vi "main.vi"() -> ()   [LabVIEW 2016]
uses:
  <vilib>/FPGAPlugInAG/myRIO-1900/niLvFpga_Open_myRIO-1900.vi
  <vilib>/rvi/interface/common/dynamic/niFpgaDynamicAddResources.vi
  <vilib>/Utility/error.llb/Error Cluster From Error Code.vi
  <vilib>/rvi/errors/niLvFpgaAdjustHostInterfaceError.vi
  <vilib>/FPGAPlugInAG/Dynamic/niLvFpga_Close_Dynamic.vi
  <vilib>/rvi/interface/nirviOpenFPGA/nirviOpenFPGA.xnode
  FPGA Bitfiles/Musicbox_FPGATarget_soundctrl_6-HSKECpU5c.lvbitx
  sound_ctrl.vi
  <vilib>/rvi/interface/nirviReadWriteControl/nirviReadWriteControl.xnode
  <vilib>/rvi/interface/nirviCloseFPGA/nirviCloseFPGA.xnode
  NiFpgaLv.dll
  <vilib>/rvi/interface/Simulation/niFpgaSimulationCallBeginRW.vi
panel:
  out "Chosen frequency":dbl
  in  "Combine frequencies":bool
  out "Saved Frequency":dbl
  in  "Add Button":bool
  out "Current Frequency":dbl
  out "Volume":dbl
  out "flag":bool
  out "index":dbl
  out "z":dbl
  out "y":dbl
  out "x":dbl
  in  "stop":bool
  out "1":string
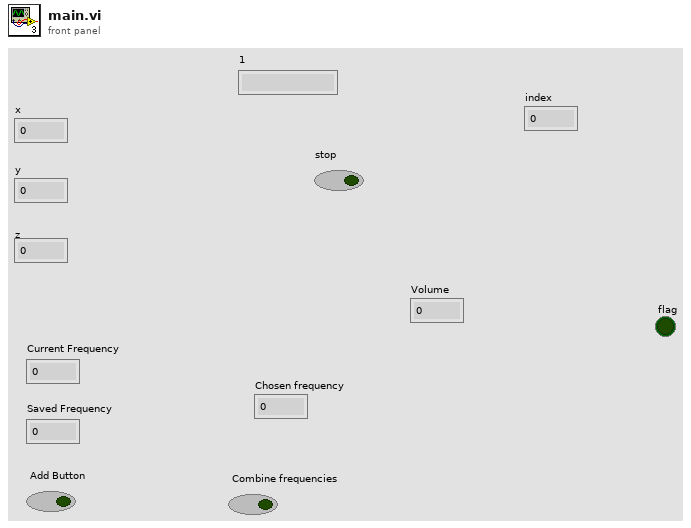
[diagram p1: front panel]
types:
  T1 = enum16{"1", "volume_+", "volume_-", "frequency+", "frequency-", "note1_selec", "note2_selec", "idle 2", "idle 3"}
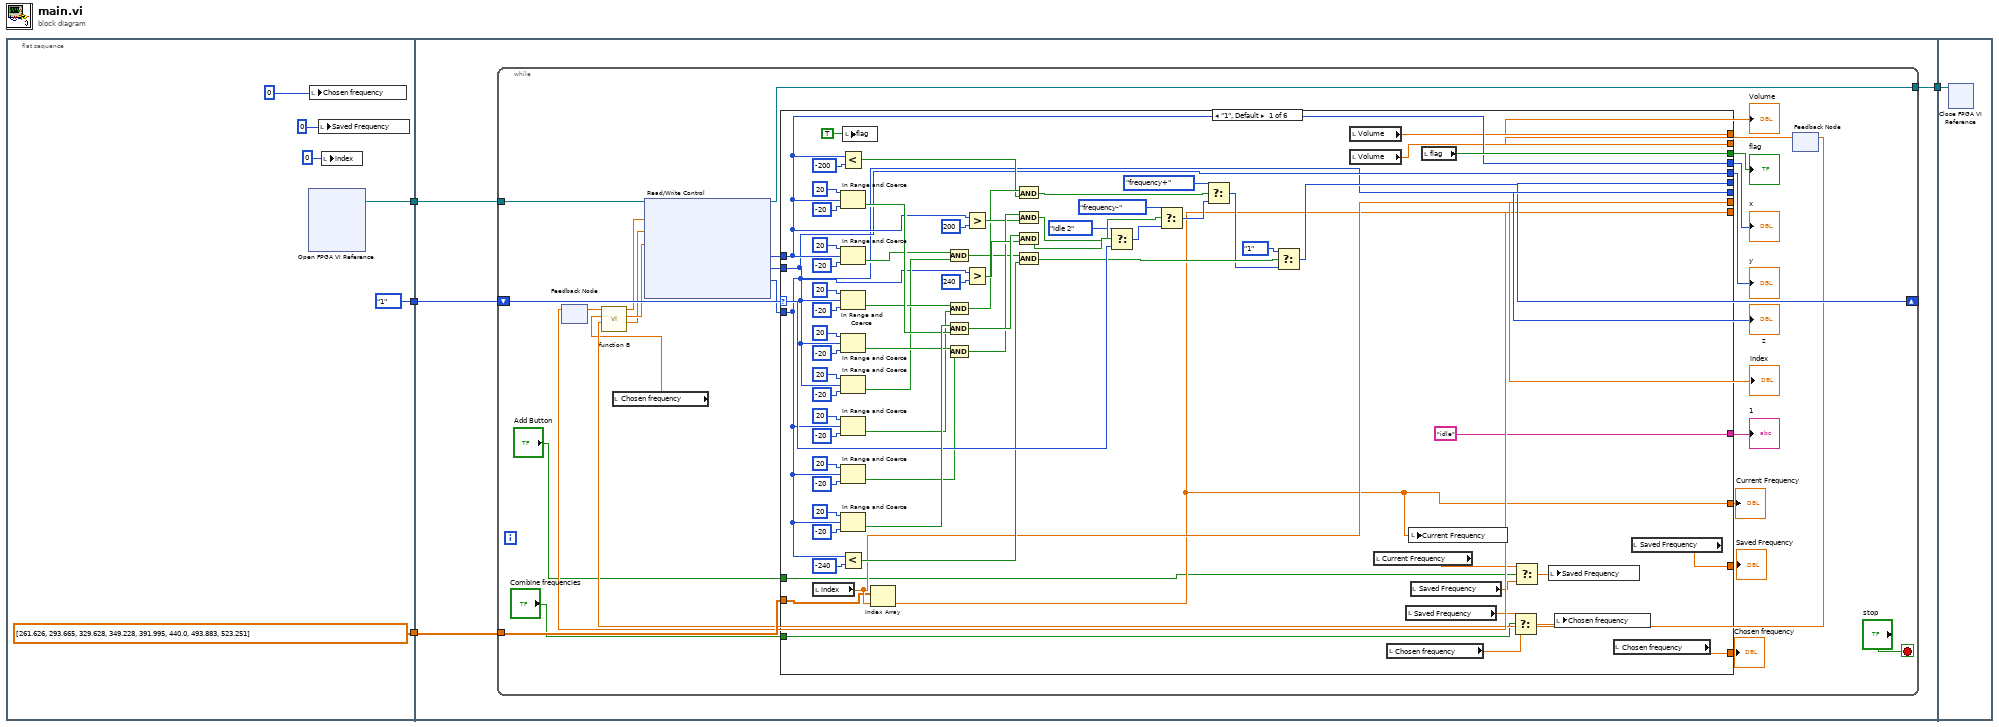
[diagram p0: block diagram]
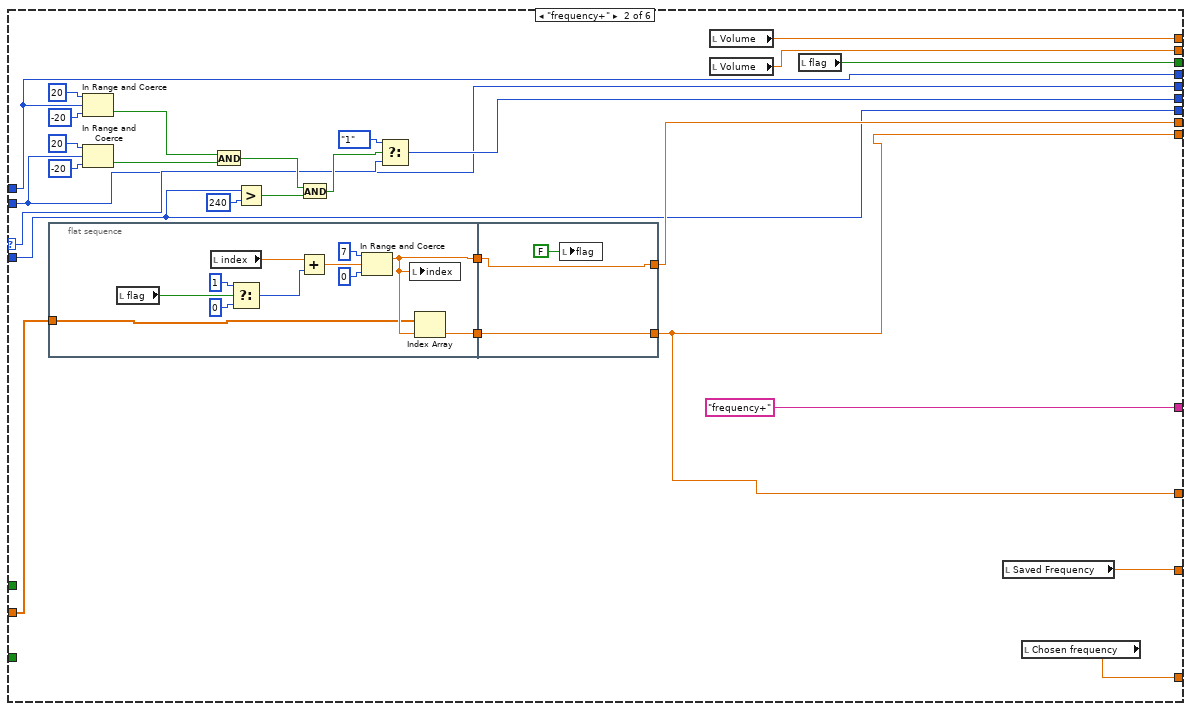
[diagram p2: hidden frame]
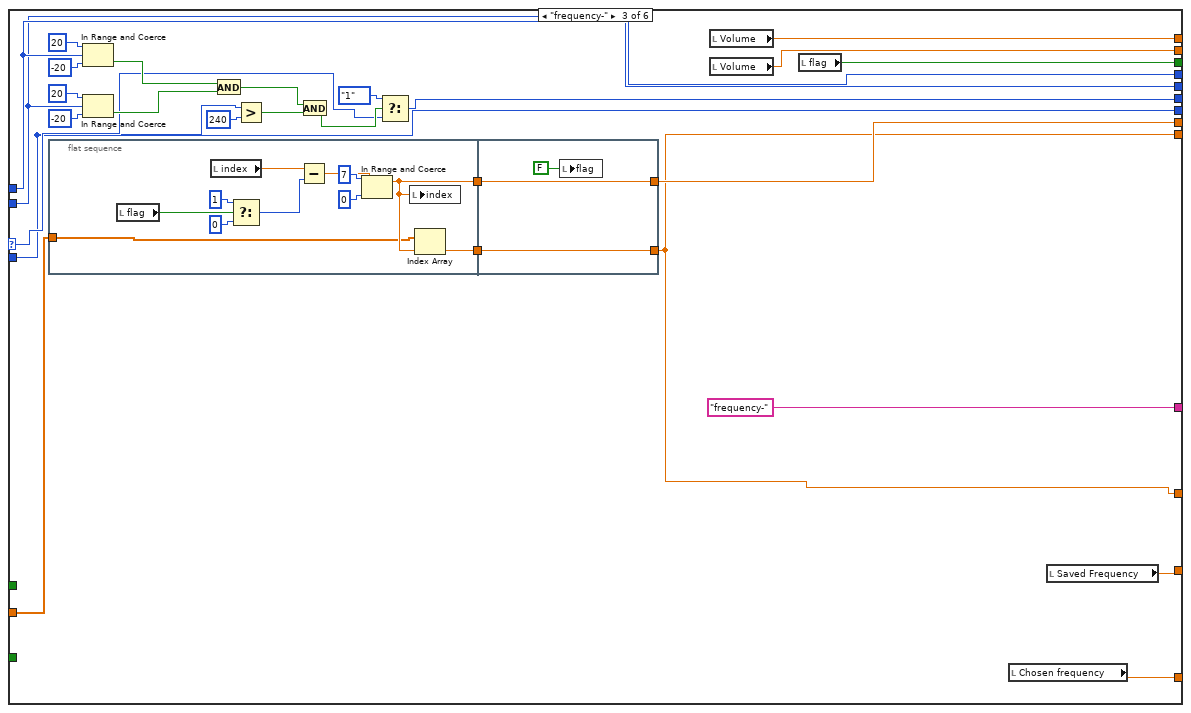
[diagram p3: hidden frame]
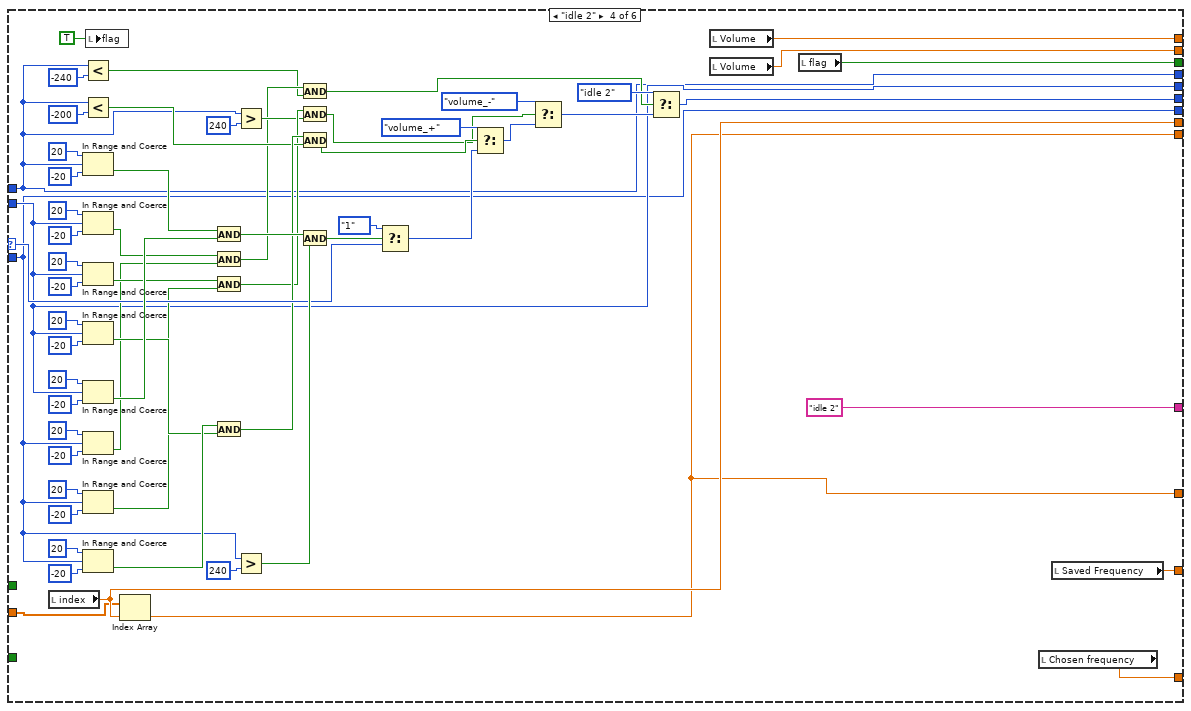
[diagram p4: hidden frame]
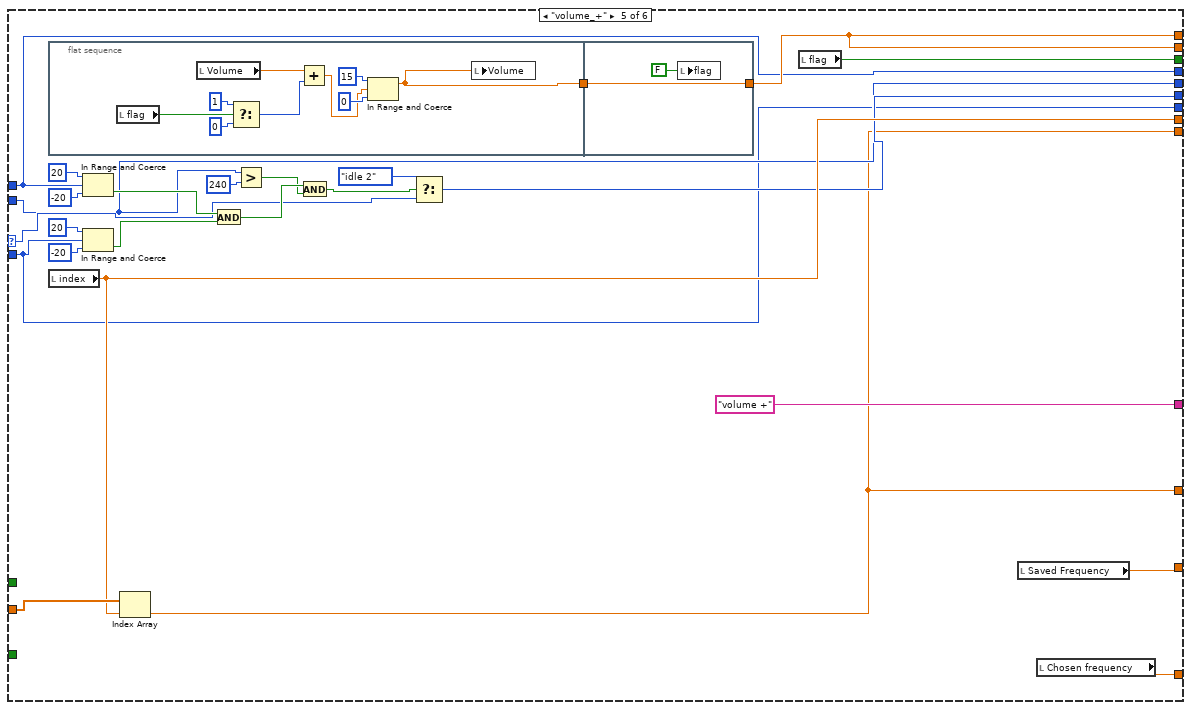
[diagram p5: hidden frame]
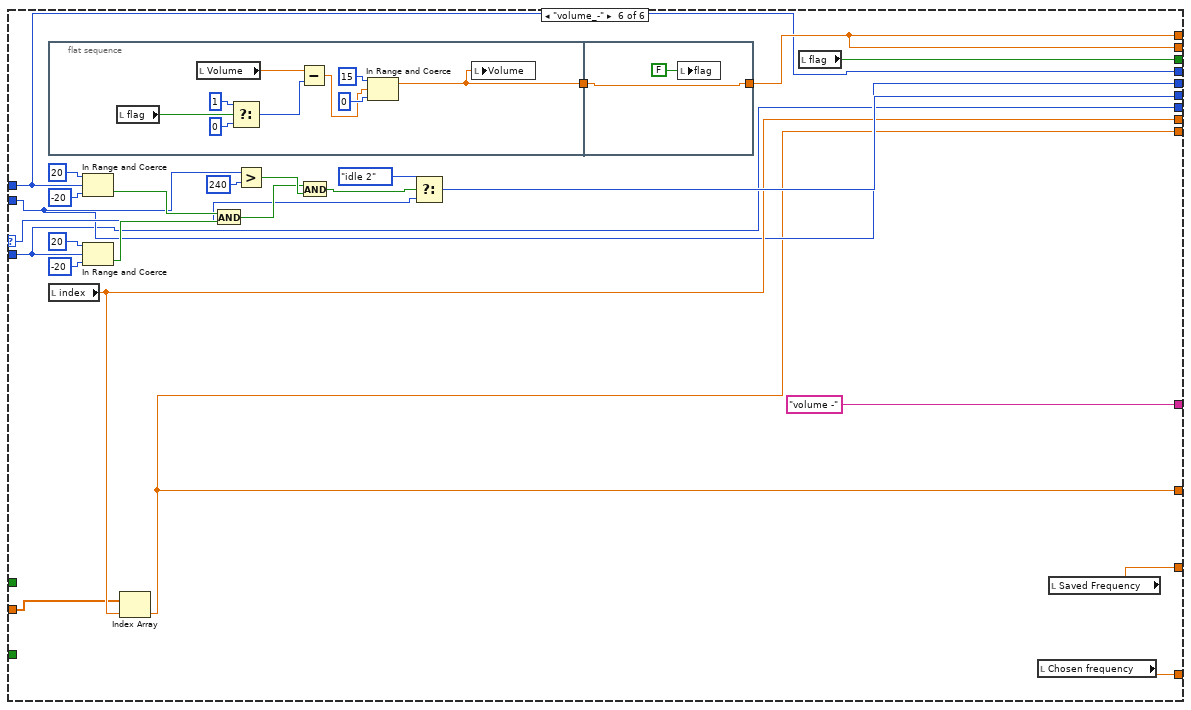
[diagram p6: hidden frame]
diagram:
  n1 = flat-sequence {
    tunnel: [w9] -> w3
    tunnel: [T1."1"] -> w2
    tunnel: [dbl[] [261.626, 293.665, 329.628, 349.228, 391.995, 440.0, 493.883, 523.251]] -> w1
    tunnel: [w14] -> w4
    tunnel: w3 -> [w13]
    tunnel: w2 -> [w12]
    tunnel: w1 -> [w11]
    tunnel: w4 -> [w329]
    frame #0 {
      n2 = xnode "Open FPGA VI Reference"() -> ("FPGA VI Reference Out"=w9:refnum<k20>)  [unwired: 2 in, 1 out]
      n3 = local write "Chosen frequency"(0) -> ()
      n4 = local write "Saved Frequency"(0) -> ()
      n5 = local write "index"(0) -> ()
    }
    frame #1 {
      n6 = while {
        shift-right: [w36] -> _
        shift-left: w12 -> [w37]
        tunnel: [w27] -> w14
        tunnel: w13 -> [w26]
        tunnel: w11 -> [w25]
        stop <- "stop" stop-if-true
        n7 = feedback #1() -> (w23:dbl)  [unwired: 1 in]
        n8 = local read "Chosen frequency"() -> (w16:dbl)
        n9 = feedback #2() -> (w20:dbl)  [unwired: 1 in]
        n10 = call "function B.vi"("frequency 1"=w23, "frequency 2"=w16, "volume"=w20) -> ("Frequency Indicator"=w30:dbl, "Frequency Indicator 2"=w29:dbl, "Volume Indicator"=w28:dbl)  [unwired: 5 in]
        n11 = xnode ("Read/Write Control")("FPGA VI Reference In"=w26, "frequency (periods/tick)"=w30, "Volume"=w28, "frequency (periods/tick) 2"=w29) -> ("FPGA VI Reference Out"=w27:refnum<k20>, "AccelerationX"=w33:i16, "AccelerationY"=w32:i16, "AccelerationZ"=w31:i16)  [unwired: 2 in, 1 out]
        n12 = case shown="\"1\", Default" w37 {
          selector: w37 -> [w101 w125 w166 w246 w262 w301]
          tunnel: ["idle" "frequency+" "frequency-" "idle 2" "volume +" "volume -"] -> w42
          tunnel: [w60 w120 w161 w199 w264 w299] -> w40
          tunnel: [w59 w119 w160 w205 w261 w297] -> w39
          tunnel: [w58 w118 w159 w198 w260 w296] -> w38
          tunnel: [w64 w123 w164 w208 w263 w304] -> w36
          tunnel: [w57 w138 w177 w204 w278 w303] -> w35
          tunnel: [w62 w122 w163 w207 w277 w298] -> w34
          tunnel: w33 -> [w60 w120 w161 w199 w264 w299]
          tunnel: w32 -> [w59 w119 w160 w205 w261 w297]
          tunnel: w31 -> [w58 w118 w159 w198 w260 w296]
          tunnel: w25 -> [w56 w121 w162 w203 w279 w302]
          tunnel: [w53 w115 w156 w197 w259 w295] -> w24
          tunnel: [w55 w116 w158 w201 w280 w300] -> w22
          tunnel: [w54 w117 w157 w202 w280 w300] -> w21
          tunnel: [w53 w115 w156 w197 w259 w295] -> w19
          tunnel: [w49 w114 w155 w196 w258 w294] -> _
          tunnel: "Add Button" -> [w48 _ _ _ _ _]
          tunnel: "Combine frequencies" -> [w47 _ _ _ _ _]
          tunnel: [w44 w113 w154 w195 w257 w293] -> w15
          frame "1", Default {
            n13 = local read "index"() -> (w57:dbl)
            n14 = Less?(x=w60, y=-200) -> (x < y?=w83:bool)
            n15 = In Range and Coerce(upper limit=20, x=w60, lower limit=-20) -> (In Range?=w105:bool)  [unwired: 1 out]
            n16 = In Range and Coerce(upper limit=20, x=w60, lower limit=-20) -> (In Range?=w72:bool)  [unwired: 1 out]
            n17 = In Range and Coerce(upper limit=20, x=w59, lower limit=-20) -> (In Range?=w86:bool)  [unwired: 1 out]
            n18 = In Range and Coerce(upper limit=20, x=w59, lower limit=-20) -> (In Range?=w96:bool)  [unwired: 1 out]
            n19 = In Range and Coerce(upper limit=20, x=w59, lower limit=-20) -> (In Range?=w71:bool)  [unwired: 1 out]
            n20 = In Range and Coerce(upper limit=20, x=w58, lower limit=-20) -> (In Range?=w85:bool)  [unwired: 1 out]
            n21 = In Range and Coerce(upper limit=20, x=w58, lower limit=-20) -> (In Range?=w95:bool)  [unwired: 1 out]
            n22 = In Range and Coerce(upper limit=20, x=w58, lower limit=-20) -> (In Range?=w106:bool)  [unwired: 1 out]
            n23 = Less?(x=w58, y=-240) -> (x < y?=w69:bool)
            n24 = local write "flag"(TRUE) -> ()
            n25 = Index Array(array=w56, index=w57) -> (element=w53:dbl)
            n26 = And(x=w72, y=w71) -> (x .and. y?=w70:bool)
            n27 = And(x=w86, y=w85) -> (x .and. y?=w84:bool)
            n28 = And(x=w106, y=w105) -> (x .and. y?=w104:bool)
            n29 = And(x=w96, y=w95) -> (x .and. y?=w94:bool)
            n30 = Greater?(x=w60, y=200) -> (0:w93:bool)
            n31 = Greater?(x=w59, y=240) -> (0:w103:bool)
            n32 = And(x=w84, y=w83) -> (x .and. y?=w81:bool)
            n33 = And(x=w94, y=w93) -> (x .and. y?=w92:bool)
            n34 = And(x=w104, y=w103) -> (x .and. y?=w102:bool)
            n35 = And(x=w70, y=w69) -> (x .and. y?=w66:bool)
            n36 = Select(t=T1."idle 2", s=w102, f=w101) -> (s? t:f=w91:T1)
            n37 = Select(t=T1."frequency-", s=w92, f=w91) -> (s? t:f=w80:T1)
            n38 = Select(t=T1."frequency+", s=w81, f=w80) -> (s? t:f=w65:T1)
            n39 = Select(t=T1."1", s=w66, f=w65) -> (s? t:f=w64:T1)
            n40 = local read "Volume"() -> (w55:dbl)
            n41 = local read "Volume"() -> (w54:dbl)
            n42 = local read "Current Frequency"() -> (w51:dbl)
            n43 = local read "Chosen frequency"() -> (w43:dbl)
            n44 = local read "Saved Frequency"() -> (w46:dbl)
            n45 = local write "Current Frequency"(w53) -> ()
            n46 = local read "Saved Frequency"() -> (w52:dbl)
            n47 = local read "flag"() -> (w62:bool)
            n48 = Select(t=w46, s=w47, f=w43) -> (s? t:f=w45:dbl)
            n49 = Select(t=w51, s=w48, f=w52) -> (s? t:f=w50:dbl)
            n50 = local write "Saved Frequency"(w50) -> ()
            n51 = local write "Chosen frequency"(w45) -> ()
            n52 = local read "Chosen frequency"() -> (w44:dbl)
            n53 = local read "Saved Frequency"() -> (w49:dbl)
          }
          frame "frequency+" {
            n54 = flat-sequence {
              tunnel: [w150] -> w137
              tunnel: [w141] -> w136
              tunnel: w121 -> [w140]
              tunnel: [w152] -> w138
              tunnel: [w153] -> w115
              tunnel: w137 -> [w153]
              tunnel: w136 -> [w152]
              frame #0 {
                n55 = local read "flag"() -> (w145:bool)
                n56 = local read "index"() -> (w149:dbl)
                n57 = Select(t=1, s=w145, f=0) -> (s? t:f=w146:i32)
                n58 = Add(x=w149, y=w146) -> (x+y=w142:dbl)
                n59 = In Range and Coerce(upper limit=7, x=w142, lower limit=0) -> (coerced(x)=w141:dbl)  [unwired: 1 out]
                n60 = local write "index"(w141) -> ()
                n61 = Index Array(array=w140, index=w141) -> (element=w150:dbl)
              }
              frame #1 {
                n62 = local write "flag"(FALSE) -> ()
              }
            }
            n63 = In Range and Coerce(upper limit=20, x=w120, lower limit=-20) -> (In Range?=w130:bool)  [unwired: 1 out]
            n64 = In Range and Coerce(upper limit=20, x=w119, lower limit=-20) -> (In Range?=w129:bool)  [unwired: 1 out]
            n65 = And(x=w130, y=w129) -> (x .and. y?=w128:bool)
            n66 = Greater?(x=w118, y=240) -> (0:w127:bool)
            n67 = And(x=w128, y=w127) -> (x .and. y?=w126:bool)
            n68 = Select(t=T1."1", s=w126, f=w125) -> (s? t:f=w123:T1)
            n69 = local read "Volume"() -> (w116:dbl)
            n70 = local read "Volume"() -> (w117:dbl)
            n71 = local read "flag"() -> (w122:bool)
            n72 = local read "Saved Frequency"() -> (w114:dbl)
            n73 = local read "Chosen frequency"() -> (w113:dbl)
          }
          frame "frequency-" {
            n74 = flat-sequence {
              tunnel: [w191] -> w179
              tunnel: [w182] -> w178
              tunnel: w162 -> [w181]
              tunnel: [w193] -> w177
              tunnel: [w194] -> w156
              tunnel: w179 -> [w194]
              tunnel: w178 -> [w193]
              frame #0 {
                n75 = local read "flag"() -> (w188:bool)
                n76 = local read "index"() -> (w187:dbl)
                n77 = Select(t=1, s=w188, f=0) -> (s? t:f=w186:i32)
                n78 = Subtract(x=w187, y=w186) -> (x-y=w183:dbl)
                n79 = In Range and Coerce(upper limit=7, x=w183, lower limit=0) -> (coerced(x)=w182:dbl)  [unwired: 1 out]
                n80 = local write "index"(w182) -> ()
                n81 = Index Array(array=w181, index=w182) -> (element=w191:dbl)
              }
              frame #1 {
                n82 = local write "flag"(FALSE) -> ()
              }
            }
            n83 = In Range and Coerce(upper limit=20, x=w161, lower limit=-20) -> (In Range?=w171:bool)  [unwired: 1 out]
            n84 = In Range and Coerce(upper limit=20, x=w160, lower limit=-20) -> (In Range?=w170:bool)  [unwired: 1 out]
            n85 = And(x=w171, y=w170) -> (x .and. y?=w169:bool)
            n86 = Greater?(x=w159, y=240) -> (0:w168:bool)
            n87 = And(x=w169, y=w168) -> (x .and. y?=w167:bool)
            n88 = Select(t=T1."1", s=w167, f=w166) -> (s? t:f=w164:T1)
            n89 = local read "Volume"() -> (w158:dbl)
            n90 = local read "Volume"() -> (w157:dbl)
            n91 = local read "flag"() -> (w163:bool)
            n92 = local read "Chosen frequency"() -> (w154:dbl)
            n93 = local read "Saved Frequency"() -> (w155:dbl)
          }
          frame "idle 2" {
            n94 = local read "index"() -> (w204:dbl)
            n95 = Less?(x=w199, y=-240) -> (x < y?=w213:bool)
            n96 = Less?(x=w199, y=-200) -> (x < y?=w237:bool)
            n97 = In Range and Coerce(upper limit=20, x=w199, lower limit=-20) -> (In Range?=w251:bool)  [unwired: 1 out]
            n98 = In Range and Coerce(upper limit=20, x=w205, lower limit=-20) -> (In Range?=w216:bool)  [unwired: 1 out]
            n99 = In Range and Coerce(upper limit=20, x=w205, lower limit=-20) -> (In Range?=w227:bool)  [unwired: 1 out]
            n100 = In Range and Coerce(upper limit=20, x=w205, lower limit=-20) -> (In Range?=w239:bool)  [unwired: 1 out]
            n101 = In Range and Coerce(upper limit=20, x=w205, lower limit=-20) -> (In Range?=w250:bool)  [unwired: 1 out]
            n102 = In Range and Coerce(upper limit=20, x=w198, lower limit=-20) -> (In Range?=w215:bool)  [unwired: 1 out]
            n103 = In Range and Coerce(upper limit=20, x=w198, lower limit=-20) -> (In Range?=w226:bool)  [unwired: 1 out]
            n104 = In Range and Coerce(upper limit=20, x=w198, lower limit=-20) -> (In Range?=w240:bool)  [unwired: 1 out]
            n105 = local write "flag"(TRUE) -> ()
            n106 = Index Array(array=w203, index=w204) -> (element=w197:dbl)
            n107 = And(x=w251, y=w250) -> (x .and. y?=w249:bool)
            n108 = And(x=w216, y=w215) -> (x .and. y?=w214:bool)
            n109 = And(x=w227, y=w226) -> (x .and. y?=w225:bool)
            n110 = And(x=w240, y=w239) -> (x .and. y?=w238:bool)
            n111 = Greater?(x=w199, y=240) -> (0:w224:bool)
            n112 = Greater?(x=w198, y=240) -> (0:w248:bool)
            n113 = And(x=w214, y=w213) -> (x .and. y?=w210:bool)
            n114 = And(x=w225, y=w224) -> (x .and. y?=w222:bool)
            n115 = And(x=w238, y=w237) -> (x .and. y?=w234:bool)
            n116 = And(x=w249, y=w248) -> (x .and. y?=w247:bool)
            n117 = Select(t=T1."1", s=w247, f=w246) -> (s? t:f=w233:T1)
            n118 = Select(t=T1."volume_+", s=w234, f=w233) -> (s? t:f=w221:T1)
            n119 = Select(t=T1."volume_-", s=w222, f=w221) -> (s? t:f=w209:T1)
            n120 = Select(t=T1."idle 2", s=w210, f=w209) -> (s? t:f=w208:T1)
            n121 = local read "Volume"() -> (w201:dbl)
            n122 = local read "Volume"() -> (w202:dbl)
            n123 = local read "flag"() -> (w207:bool)
            n124 = local read "Chosen frequency"() -> (w195:dbl)
            n125 = local read "Saved Frequency"() -> (w196:dbl)
          }
          frame "volume_+" {
            n126 = flat-sequence {
              tunnel: [w282] -> w281
              tunnel: [w292] -> w280
              tunnel: w281 -> [w292]
              frame #0 {
                n127 = local read "flag"() -> (w286:bool)
                n128 = local read "Volume"() -> (w290:dbl)
                n129 = Select(t=1, s=w286, f=0) -> (s? t:f=w287:i32)
                n130 = Add(x=w290, y=w287) -> (x+y=w283:dbl)
                n131 = In Range and Coerce(upper limit=15, x=w283, lower limit=0) -> (coerced(x)=w282:dbl)  [unwired: 1 out]
                n132 = local write "Volume"(w282) -> ()
              }
              frame #1 {
                n133 = local write "flag"(FALSE) -> ()
              }
            }
            n134 = local read "index"() -> (w278:dbl)
            n135 = In Range and Coerce(upper limit=20, x=w264, lower limit=-20) -> (In Range?=w270:bool)  [unwired: 1 out]
            n136 = In Range and Coerce(upper limit=20, x=w260, lower limit=-20) -> (In Range?=w269:bool)  [unwired: 1 out]
            n137 = Index Array(array=w279, index=w278) -> (element=w259:dbl)
            n138 = And(x=w270, y=w269) -> (x .and. y?=w268:bool)
            n139 = Greater?(x=w261, y=240) -> (0:w267:bool)
            n140 = And(x=w268, y=w267) -> (x .and. y?=w266:bool)
            n141 = Select(t=T1."idle 2", s=w266, f=w262) -> (s? t:f=w263:T1)
            n142 = local read "flag"() -> (w277:bool)
            n143 = local read "Saved Frequency"() -> (w258:dbl)
            n144 = local read "Chosen frequency"() -> (w257:dbl)
          }
          frame "volume_-" {
            n145 = flat-sequence {
              tunnel: [w318] -> w317
              tunnel: [w328] -> w300
              tunnel: w317 -> [w328]
              frame #0 {
                n146 = local read "flag"() -> (w322:bool)
                n147 = local read "Volume"() -> (w326:dbl)
                n148 = Select(t=1, s=w322, f=0) -> (s? t:f=w323:i32)
                n149 = Subtract(x=w326, y=w323) -> (x-y=w319:dbl)
                n150 = In Range and Coerce(upper limit=15, x=w319, lower limit=0) -> (coerced(x)=w318:dbl)  [unwired: 1 out]
                n151 = local write "Volume"(w318) -> ()
              }
              frame #1 {
                n152 = local write "flag"(FALSE) -> ()
              }
            }
            n153 = local read "index"() -> (w303:dbl)
            n154 = In Range and Coerce(upper limit=20, x=w299, lower limit=-20) -> (In Range?=w311:bool)  [unwired: 1 out]
            n155 = In Range and Coerce(upper limit=20, x=w296, lower limit=-20) -> (In Range?=w312:bool)  [unwired: 1 out]
            n156 = Index Array(array=w302, index=w303) -> (element=w295:dbl)
            n157 = And(x=w311, y=w312) -> (x .and. y?=w313:bool)
            n158 = Greater?(x=w297, y=240) -> (0:w314:bool)
            n159 = And(x=w313, y=w314) -> (x .and. y?=w315:bool)
            n160 = Select(t=T1."idle 2", s=w315, f=w301) -> (s? t:f=w304:T1)
            n161 = local read "flag"() -> (w298:bool)
            n162 = local read "Chosen frequency"() -> (w293:dbl)
            n163 = local read "Saved Frequency"() -> (w294:dbl)
          }
        }
        "1" <- w42
        "x" <- w40
        "y" <- w39
        "z" <- w38
        "index" <- w35
        "flag" <- w34
        "Volume" <- w22
        "Current Frequency" <- w19
        "Chosen frequency" <- w15
        n164 = feedback-in #1(w24) -> ()
        n165 = feedback-in #2(w21) -> ()
      }
    }
    frame #2 {
      n166 = xnode "Close FPGA VI Reference"("FPGA VI Reference In"=w329) -> ()  [unwired: 1 in, 1 out]
    }
  }
